vi "Conf Temperature.vi"(0 "VISA Resource Name":refnum<visa-resource-name>, 1 "Transducer Type (0:TC)":T5(ring), 2 "Set/Check? (F:Set)":bool, 3 "Check Parameter (0:Units)":T4(ring), 5 "Thermocouple Configuration":T2={"Thermocouple Type (Last)"=enum."Default (Last)", "TC Rjunction (2:Int)"=enum."Internal", "Fixed Rjunction Temp (0:Manual)"=enum."Manual", "TC Auto Check? (F:Don't Check)"=FALSE, "Rjunct Temp Value (0)"=0.0} {"Rjunct Temp Value (0)" min=-20.0 max=80.0 format="%.2f"}, 7 "RTD Configuration":T1={"RTD Type (2:Last)"=enum."Default (Last)", "RTD Ref Resistance (100)"=100.0} {"RTD Ref Resistance (100)" min=4.9 max=2100.0 format="%.2f"}, 9 "Thermistor Type (3:Last)":T3(ring)=enum."Default (Last)", 11 "error in (no error)":errorcluster, 12 "Channel List(empty)":string, 13 "Units (0:Celsius)":enum16{"Celsius", "Fahrenheit", "Kelvin"}(ring)) -> (4 "VISA Resource Name Out":refnum<visa-resource-name>, 8 "Configuration?":string, 15 "error out":errorcluster)   [LabVIEW 2015, in "Agilent 34970.lvlib"]
doc: "This VI configures the instrument for advanced temperature measurements.\n\nThis is an advanced measurment configuration VI. For more information on the different ways to take and configure a measurment, refer to the context help and block diagram of \"HP34970A Advanced Scan Example.vi\"."
uses:
  <instrlib>/Agilent 34970/Agilent 34970.lvlib
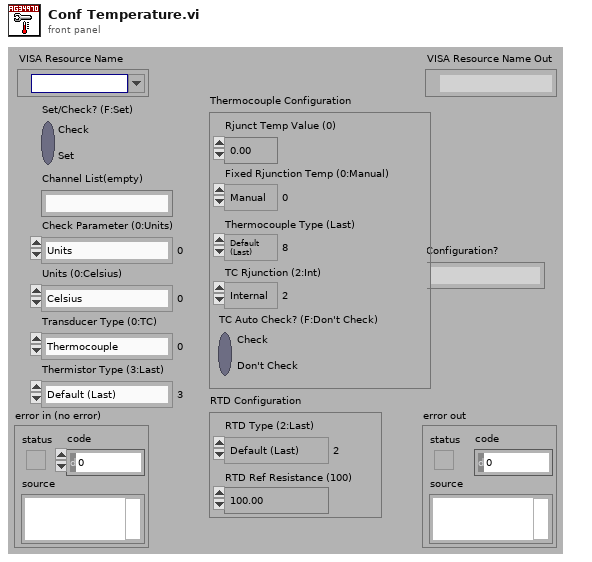
[diagram p1: front panel]
types:
  T1 = cluster{"RTD Type (2:Last)":enum16{"85", "91", "Default (Last)"}, "RTD Ref Resistance (100)":dbl}
  T2 = cluster{"Thermocouple Type (Last)":enum16{"B", "E", "J", "K", "N", "R", "S", "T", "Default (Last)"}, "TC Rjunction (2:Int)":enum16{"Fixed", "External", "Internal"}, "Fixed Rjunction Temp (0:Manual)":enum16{"Manual", "Minimum", "Maximum"}, "TC Auto Check? (F:Don't Check)":bool, "Rjunct Temp Value (0)":dbl}
  T3 = enum16{"2252", "5000", "10000", "Default (Last)"}
  T4 = enum16{"Units", "Thermocouple Type", "Rjunction Type", "Rjunction Temp", "Fixed Rjunction Temp", "Auto TC Check", "RTD Ref Resistance", "FRTD Ref Resistance"}
  T5 = enum16{"Thermocouple", "Thermistor", "RTD", "4-Wire RTD"}
  T6 = enum16{"B", "E", "J", "K", "N", "R", "S", "T", "Default (Last)"}
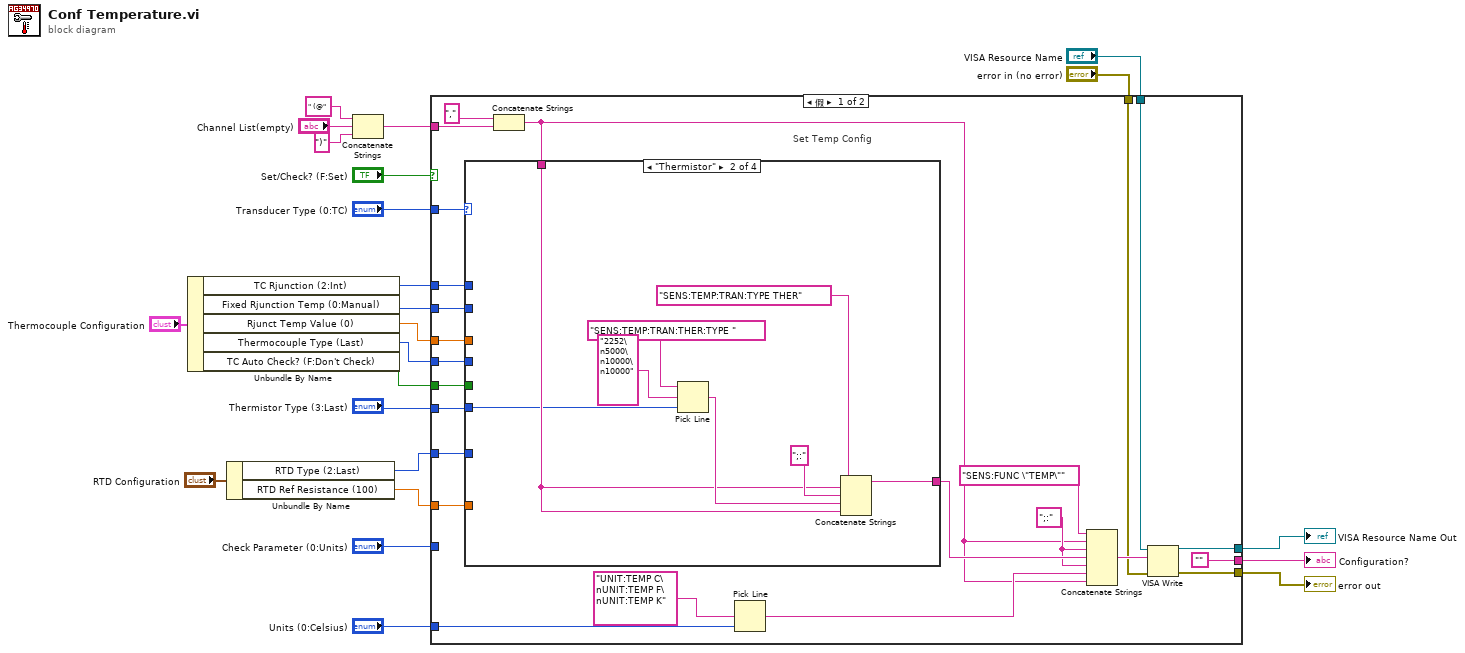
[diagram p0: block diagram]
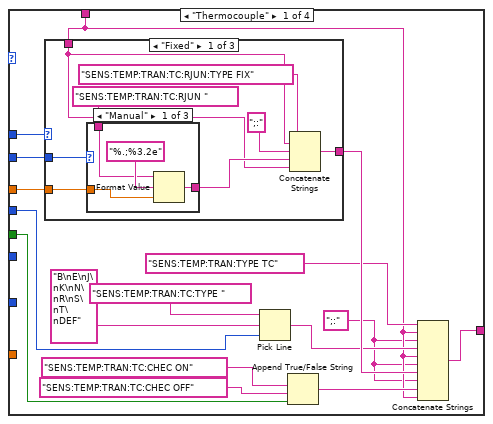
[diagram p2: hidden frame]
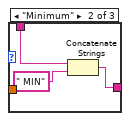
[diagram p3: hidden frame]
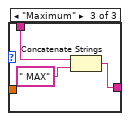
[diagram p4: hidden frame]
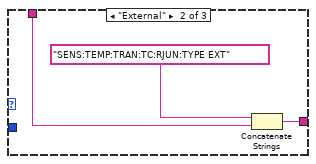
[diagram p5: hidden frame]
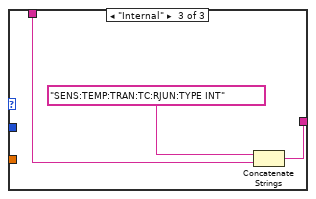
[diagram p6: hidden frame]
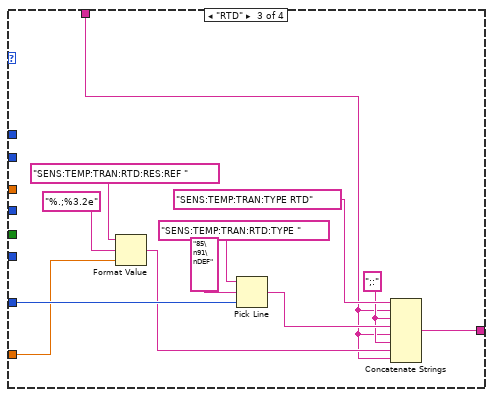
[diagram p7: hidden frame]
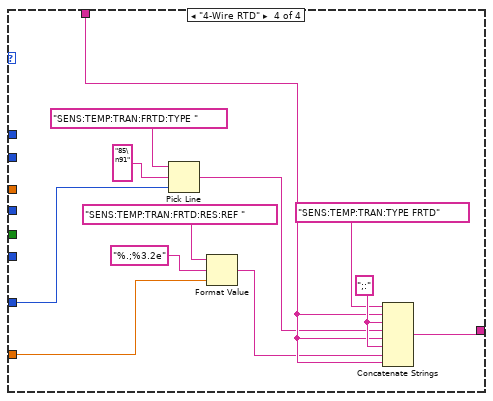
[diagram p8: hidden frame]
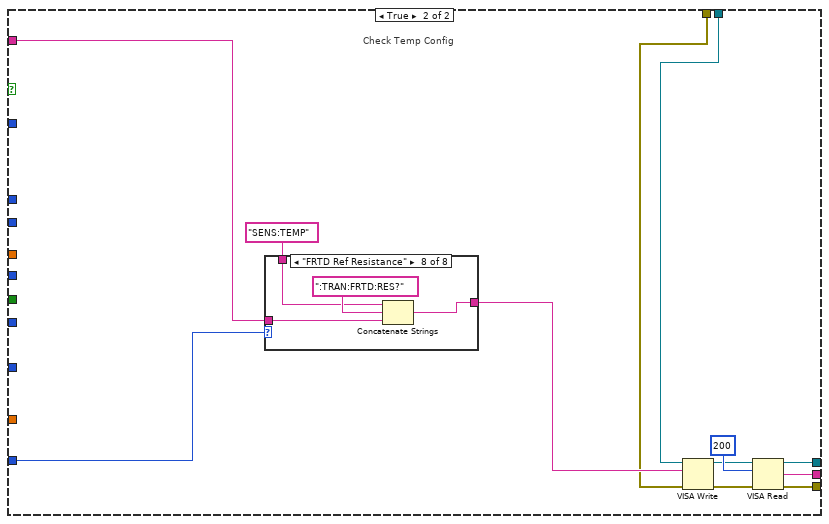
[diagram p9: hidden frame]
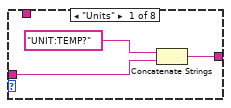
[diagram p10: hidden frame]
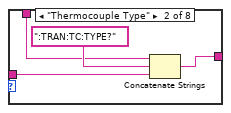
[diagram p11: hidden frame]
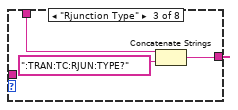
[diagram p12: hidden frame]
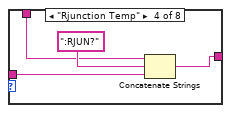
[diagram p13: hidden frame]
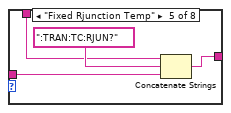
[diagram p14: hidden frame]
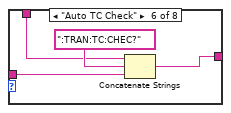
[diagram p15: hidden frame]
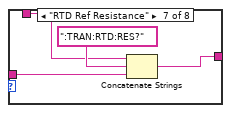
[diagram p16: hidden frame]
diagram:
  n1 = Unbundle By Name("Thermocouple Configuration") -> ("TC Rjunction (2:Int)"=w6:enum16{"Fixed", "External", "Internal"}, "Fixed Rjunction Temp (0:Manual)"=w5:enum16{"Manual", "Minimum", "Maximum"}, "Rjunct Temp Value (0)"=w4:dbl, "Thermocouple Type (Last)"=w3:T6, "TC Auto Check? (F:Don't Check)"=w12:bool)
  n2 = Unbundle By Name("RTD Configuration") -> ("RTD Type (2:Last)"=w10:enum16{"85", "91", "Default (Last)"}, "RTD Ref Resistance (100)"=w9:dbl)
  n3 = Concatenate Strings(" (@", "Channel List(empty)", ")") -> (w21:string)
  n4 = case shown="假" "Set/Check? (F:Set)" {
    tunnel: [w45 w131] -> w7
    tunnel: [w46 w128] -> w8
    tunnel: w21 -> [w43 w123]
    tunnel: ["" w129] -> w20
    tunnel: "Transducer Type (0:TC)" -> [w42 _]
    tunnel: w5 -> [w29 _]
    tunnel: w12 -> [w30 _]
    tunnel: "Thermistor Type (3:Last)" -> [w31 _]
    tunnel: w10 -> [w32 _]
    tunnel: w9 -> [w41 _]
    tunnel: "Units (0:Celsius)" -> [w39 _]
    tunnel: "Check Parameter (0:Units)" -> [_ w124]
    tunnel: w6 -> [w28 _]
    tunnel: w4 -> [w27 _]
    tunnel: w3 -> [w26 _]
    tunnel: "error in (no error)" -> [w25 w121]
    tunnel: "VISA Resource Name" -> [w24 w120]
    frame False {
      w36 = ";:"
      # "Set Temp Config"
      n5 = Concatenate Strings(",", w43) -> (w34:string)
      n6 = case shown="\"Thermistor\"" w42 {
        tunnel: w29 -> [w61 _ _ _]
        tunnel: w30 -> [w58 _ _ _]
        tunnel: w31 -> [_ w88 _ _]
        tunnel: w32 -> [_ _ w104 w115]
        tunnel: w41 -> [_ _ w102 w114]
        tunnel: w34 -> [w52 w90 w97 w111]
        tunnel: [w55 w89 w96 w108] -> w37
        tunnel: w28 -> [w50 _ _ _]
        tunnel: w27 -> [w49 _ _ _]
        tunnel: w26 -> [w48 _ _ _]
        frame "Thermocouple" {
          w51 = ";:"
          n7 = case shown="\"Fixed\"" w50 {
            tunnel: w61 -> [w71 _ _]
            tunnel: w52 -> [w66 w84 w87]
            tunnel: [w65 w82 w85] -> w57
            tunnel: w49 -> [w64 _ _]
            frame "Fixed" {
              n8 = case shown="\"Manual\"" w71 {
                tunnel: [w75 w77 w80] -> w69
                tunnel: "SENS:TEMP:TRAN:TC:RJUN " -> [w73 w76 w79]
                tunnel: w64 -> [w72 _ _]
                frame "Manual" {
                  n9 = Format Value(string ("")=w73, format string="%.;%3.2e", value (0)=w72) -> (output string=w75:string)
                }
                frame "Minimum" {
                  n10 = Concatenate Strings(w76, " MIN") -> (w77:string)
                }
                frame "Maximum" {
                  n11 = Concatenate Strings(w79, " MAX") -> (w80:string)
                }
              }
              n12 = Concatenate Strings("SENS:TEMP:TRAN:TC:RJUN:TYPE FIX", w66, ";:", w69, w66) -> (w65:string)
            }
            frame "External" {
              n13 = Concatenate Strings("SENS:TEMP:TRAN:TC:RJUN:TYPE EXT", w84) -> (w82:string)
            }
            frame "Internal" {
              n14 = Concatenate Strings("SENS:TEMP:TRAN:TC:RJUN:TYPE INT", w87) -> (w85:string)
            }
          }
          n15 = Pick Line(string ("")="SENS:TEMP:TRAN:TC:TYPE ", multi-line string="B\nE\nJ\nK\nN\nR\nS\nT\nDEF", line index=w48) -> (output string=w54:string)
          n16 = Append True/False String(1:w58, 2:"SENS:TEMP:TRAN:TC:CHEC OFF" ("multi-line string"), 3:"SENS:TEMP:TRAN:TC:CHEC ON" ("multi-line string")) -> (0:w56:string)  [unwired: 1 in]
          n17 = Concatenate Strings("SENS:TEMP:TRAN:TYPE TC", w52, w51, w54, w52, w51, w57, w51, w56, w52) -> (w55:string)
        }
        frame "Thermistor" {
          n18 = Pick Line(string ("")="SENS:TEMP:TRAN:THER:TYPE ", multi-line string="2252\n5000\n10000\n10000", line index=w88) -> (output string=w91:string)
          n19 = Concatenate Strings("SENS:TEMP:TRAN:TYPE THER", w90, ";:", w91, w90) -> (w89:string)
        }
        frame "RTD" {
          w99 = ";:"
          n20 = Format Value(string ("")="SENS:TEMP:TRAN:RTD:RES:REF ", format string="%.;%3.2e", value (0)=w102) -> (output string=w98:string)
          n21 = Pick Line(string ("")="SENS:TEMP:TRAN:RTD:TYPE ", multi-line string="85\n91\nDEF", line index=w104) -> (output string=w100:string)
          n22 = Concatenate Strings("SENS:TEMP:TRAN:TYPE RTD", w97, w99, w100, w97, w99, w98, w97) -> (w96:string)
        }
        frame "4-Wire RTD" {
          w113 = ";:"
          n23 = Pick Line(string ("")="SENS:TEMP:TRAN:FRTD:TYPE ", multi-line string="85\n91", line index=w115) -> (output string=w110:string)
          n24 = Format Value(string ("")="SENS:TEMP:TRAN:FRTD:RES:REF ", format string="%.;%3.2e", value (0)=w114) -> (output string=w109:string)
          n25 = Concatenate Strings("SENS:TEMP:TRAN:TYPE FRTD", w111, w113, w110, w111, w113, w109, w111) -> (w108:string)
        }
      }
      n26 = Pick Line(multi-line string="UNIT:TEMP C\nUNIT:TEMP F\nUNIT:TEMP K", line index=w39) -> (output string=w35:string)  [unwired: 1 in]
      n27 = Concatenate Strings("SENS:FUNC \"TEMP\"", w34, w36, w37, w36, w35, w34) -> (w33:string)
      n28 = VISA Write(VISA resource name=w24, write buffer=w33, error in (no error)=w25) -> (VISA resource name out=w46:refnum<visa-resource-name>, error out=w45:errorcluster)  [unwired: 1 out]
    }
    frame True {
      # "Check Temp Config"
      n29 = case shown="\"FRTD Ref Resistance\"" w124 {
        tunnel: "SENS:TEMP" -> [_ w137 w141 w144 w148 w152 w156 w160]
        tunnel: [w133 w136 w139 w143 w147 w151 w155 w159] -> w122
        tunnel: w123 -> [w132 w135 _ w142 w146 w150 w154 w158]
        frame "Units" {
          n30 = Concatenate Strings("UNIT:TEMP?", w132) -> (w133:string)
        }
        frame "Thermocouple Type" {
          n31 = Concatenate Strings(w137, ":TRAN:TC:TYPE?", w135) -> (w136:string)
        }
        frame "Rjunction Type" {
          n32 = Concatenate Strings(w141, ":TRAN:TC:RJUN:TYPE?") -> (w139:string)
        }
        frame "Rjunction Temp" {
          n33 = Concatenate Strings(w144, ":RJUN?", w142) -> (w143:string)
        }
        frame "Fixed Rjunction Temp" {
          n34 = Concatenate Strings(w148, ":TRAN:TC:RJUN?", w146) -> (w147:string)
        }
        frame "Auto TC Check" {
          n35 = Concatenate Strings(w152, ":TRAN:TC:CHEC?", w150) -> (w151:string)
        }
        frame "RTD Ref Resistance" {
          n36 = Concatenate Strings(w156, ":TRAN:RTD:RES?", w154) -> (w155:string)
        }
        frame "FRTD Ref Resistance" {
          n37 = Concatenate Strings(w160, ":TRAN:FRTD:RES?", w158) -> (w159:string)
        }
      }
      n38 = VISA Write(VISA resource name=w120, write buffer=w122, error in (no error)=w121) -> (VISA resource name out=w127:refnum<visa-resource-name>, error out=w126:errorcluster)  [unwired: 1 out]
      n39 = VISA Read(VISA resource name=w127, byte count=u32 200 ("byte count (0)"), error in (no error)=w126) -> (VISA resource name out=w128:refnum<visa-resource-name>, read buffer=w129:string, error out=w131:errorcluster)  [unwired: 1 out]
    }
  }
  "Configuration?" <- w20
  "VISA Resource Name Out" <- w8
  "error out" <- w7
